vi "main.vi"() -> ()   [LabVIEW 2023]
uses:
  <vilib>/Instr/_visa.llb/VISA Configure Serial Port (Instr).vi
panel:
  in  "Tab Control":enum32{"OSCILOSCOPIO", ""}(tab)
  in  "Escala 1 / Escala 2":bool
  in  "Escala":dbl(knob) scale=-30.0..30.0
  in  "Canal 2":bool
  in  "Canal 1":bool
  out "Osciloscopio":dynamicdata(graph)
  in  "Puerto Serie":refnum<visa-resource-name>
  in  "stop":bool
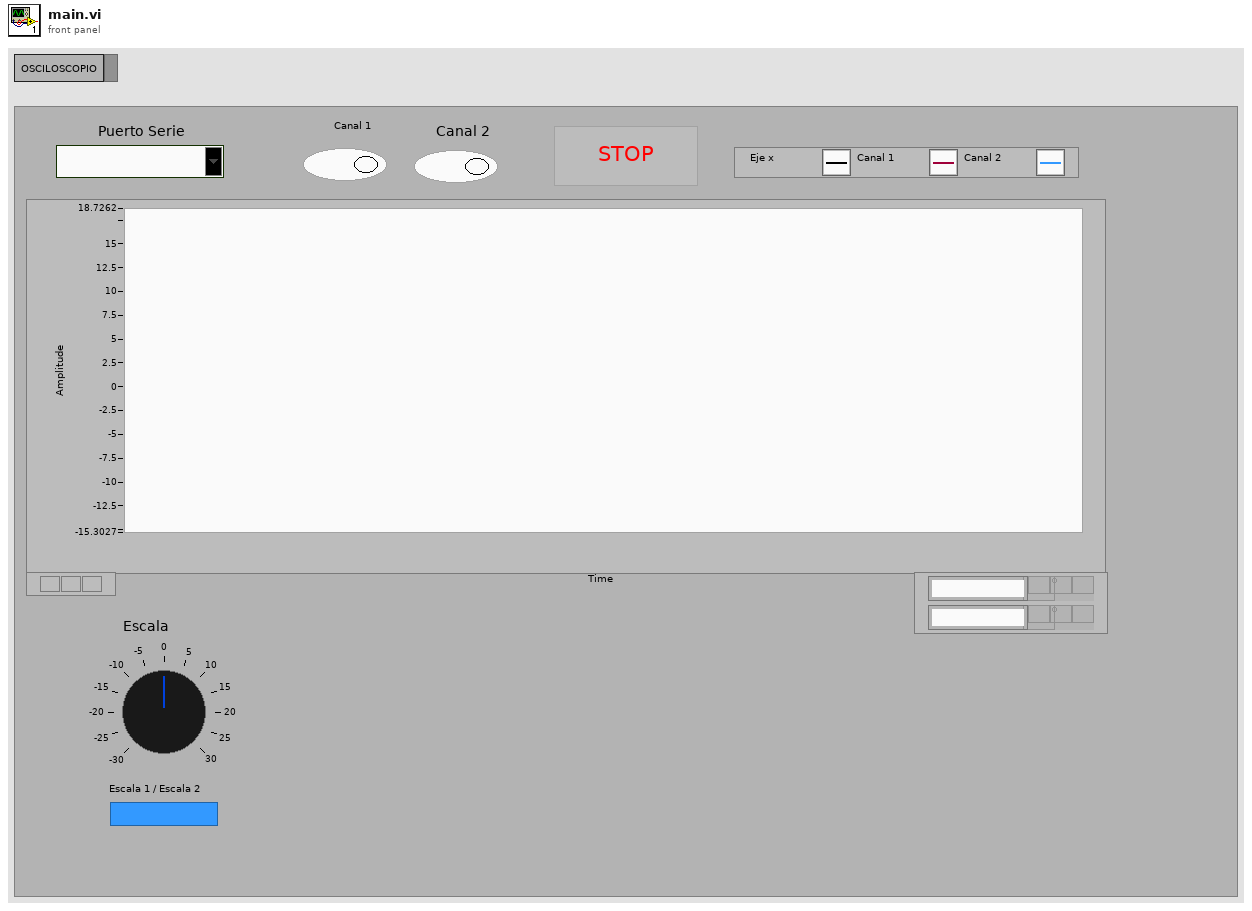
[diagram p1: front panel]
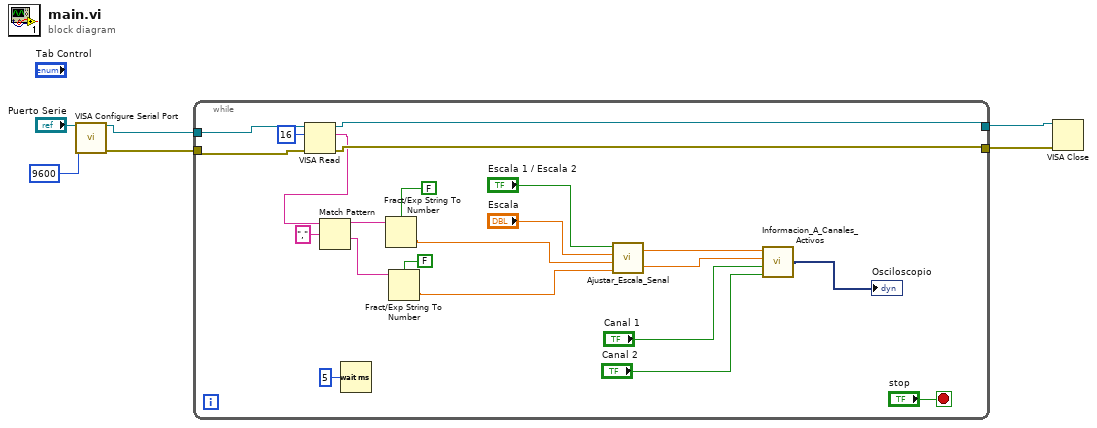
[diagram p0: block diagram]
diagram:
  n1 = call-poly "VISA Configure Serial Port"("VISA resource name"="Puerto Serie", "baud rate (9600)"=u32 9600) -> ("VISA resource name out"=w5:refnum<visa-resource-name>, "error out"=w4:errorcluster)  [unwired: 12 in]
  n2 = while {
    tunnel: w5 -> [w28]
    tunnel: w4 -> [w27]
    tunnel: [w26] -> w3
    tunnel: [w25] -> w2
    stop <- "stop" stop-if-true
    n3 = VISA Read(VISA resource name=w28, byte count=u32 16, error in (no error)=w27) -> (VISA resource name out=w26:refnum<visa-resource-name>, read buffer=w20:string, error out=w25:errorcluster)  [unwired: 1 out]
    n4 = Match Pattern(string=w20, regular expression=",") -> (before substring=w18:string, after substring=w17:string)  [unwired: 1 in, 2 out]
    n5 = Wait (ms)(milliseconds to wait=u32 5) -> ()  [unwired: 1 out]
    n6 = Fract/Exp String To Number(use system decimal point (T)=FALSE, string=w18) -> (number=w10:dbl)  [unwired: 2 in, 1 out]
    n7 = Fract/Exp String To Number(use system decimal point (T)=FALSE, string=w17) -> (number=w9:dbl)  [unwired: 2 in, 1 out]
    n8 = call "Ajustar_Escala_Senal.vi"("Data_Canal_2"=w9, "Data_Canal_1"=w10, "Escala"="Escala", "Tipo_Canal"="Escala 1 / Escala 2") -> ("Data_Canal_2"=w7:dbl, "Data_Canal_1"=w8:dbl)
    n9 = call "Informacion_A_Canales_Activos.vi"("Canal_Activo_2"="Canal 2", "Canal_Activo_1"="Canal 1", "Data_Canal_2"=w7, "Data_Canal_1"=w8) -> ("Data"=→"Osciloscopio":dynamicdata)
  }
  n10 = VISA Close(VISA resource name=w3, error in (no error)=w2) -> ()  [unwired: 1 out]
